vi "Retest.vi"() -> ()   [LabVIEW 2018]
uses:
  Ctl Main/Global Variable.vi
panel:
  in  "Retest Cnt":dbl
  in  "Debugging":bool
  in  "Parameters":string[](array[string])
  in  "Retest ON":bool
  # "Retest"
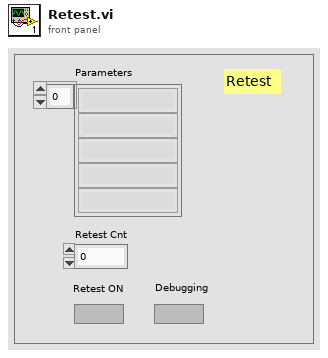
[diagram p1: front panel]
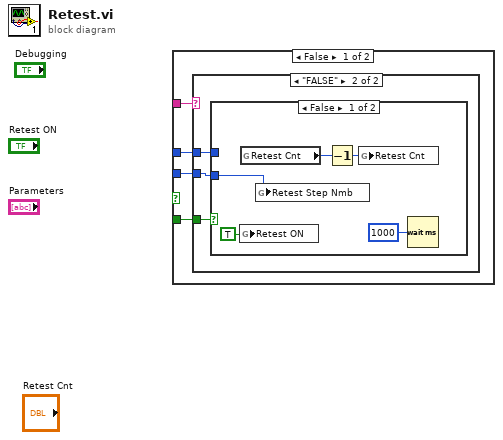
[diagram p0: block diagram]
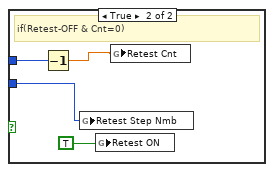
[diagram p3: hidden frame]
diagram:
  n1 = case shown="False" {
    selector: _ -> [_ _]
    tunnel: _ -> [w4 _]
    tunnel: _ -> [w1 _]
    tunnel: _ -> [w3 _]
    tunnel: _ -> [w2 _]
    frame False {
      n2 = case shown="\"FALSE\"" w4 {
        tunnel: w1 -> [_ w5]
        tunnel: w3 -> [_ w7]
        tunnel: w2 -> [_ w6]
        frame "Idle", Default {
        }
        frame "FALSE" {
          n3 = case shown="False" w5 {
            tunnel: w7 -> [_ w14]
            tunnel: w6 -> [w9 w16]
            frame False {
              n4 = global write "Global Variable.vi" "Retest ON"(TRUE ("Retest ON")) -> ()
              n5 = global read "Global Variable.vi" "Retest Cnt"() -> (w12:i16)
              n6 = global write "Global Variable.vi" "Retest Step Nmb"(w9) -> ()
              n7 = Decrement(x=w12) -> (x-1=w11:i16)
              n8 = global write "Global Variable.vi" "Retest Cnt"(w11) -> ()
              n9 = Wait (ms)(milliseconds to wait=u32 1000) -> ()  [unwired: 1 out]
            }
            frame True {
              # "if(Retest-OFF & Cnt=0)"
              n10 = Decrement(x=w14) -> (x-1=w13:dbl)
              n11 = global write "Global Variable.vi" "Retest Step Nmb"(w16) -> ()
              n12 = global write "Global Variable.vi" "Retest ON"(TRUE ("Retest ON")) -> ()
              n13 = global write "Global Variable.vi" "Retest Cnt"(w13) -> ()
            }
          }
        }
      }
    }
    frame True {
    }
  }
